vi "parse_colorRGBA.vi"(4 "error in":errorcluster, 7 "msg in":string) -> (0 "error out":errorcluster, 2 "Color RGBA":cluster{"R":dbl, "G":dbl, "A":dbl, "B":dbl}, 3 "msg out":string)   [LabVIEW 2015]
uses:
  subs/parse_float32_scalar.vi
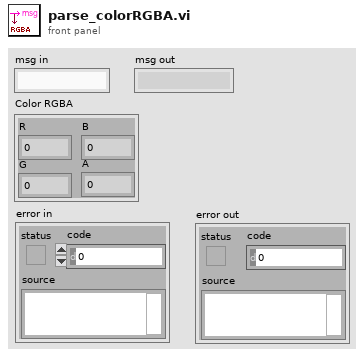
[diagram p1: front panel]
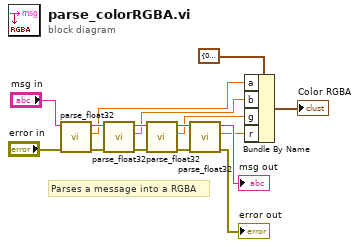
[diagram p0: block diagram]
diagram:
  # "Parses a message into a RGBA"
  n1 = call-poly "parse_float32.vi"("error in"="error in", "msg in"="msg in") -> ("error out"=w8:errorcluster, "number"=w4:sgl, "msg out"=w13:string)  [unwired: 3 in]
  n2 = call-poly "parse_float32.vi"("error in"=w8, "msg in"=w13) -> ("error out"=w7:errorcluster, "number"=w3:sgl, "msg out"=w12:string)  [unwired: 3 in]
  n3 = call-poly "parse_float32.vi"("error in"=w7, "msg in"=w12) -> ("error out"=w6:errorcluster, "number"=w2:sgl, "msg out"=w11:string)  [unwired: 3 in]
  n4 = call-poly "parse_float32.vi"("error in"=w6, "msg in"=w11) -> ("error out"=→"error out":errorcluster, "number"=w1:sgl, "msg out"=→"msg out":string)  [unwired: 3 in]
  n5 = Bundle By Name(cluster=cluster{"a":dbl, "b":dbl, "g":dbl, "r":dbl} {"a"=0.0, "b"=0.0, "g"=0.0, "r"=0.0} ("Quaternion"), "a"=w4, "b"=w3, "g"=w2, "r"=w1) -> (→"Color RGBA":cluster{"a":dbl, "b":dbl, "g":dbl, "r":dbl})
